vi "round val.vi"(1 "num in":dbl) -> (0 "num out":dbl)   [LabVIEW 2012]
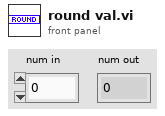
[diagram p1: front panel]
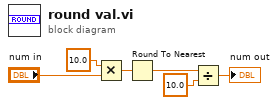
[diagram p0: block diagram]
diagram:
  n1 = Multiply(x=10.0, y="num in") -> (x*y=w2:dbl)
  n2 = Round To Nearest(number=w2) -> (nearest integer value=w1:dbl)
  n3 = Divide(x=w1, y=10.0) -> (x/y=→"num out":dbl)
